vi "App - FileSync Example.vi"() -> ()   [LabVIEW 2020]
uses:
  <userlib>/_NEVSTOP/Communicable State Machine(CSM)/addons/MassData-Parameter/Utility/Def-MassData Status Indicator(Vertical).ctl
  Protocol/Base/Def-FileSyncConfig.ctl
  CSM-FileSync.lvlib
  Protocol/Base/Protocol.lvclass
  Protocol/FTP/FTPProtocol.lvclass
  <userlib>/_NEVSTOP/Communicable State Machine(CSM)/Communicable State Machine.lvlib
  D:/NEVSTOP-LAB-Development/csm-modsets/CSM-ModSets-FileSync/Protocol/Base/Protocol.lvclass
panel:
  in  "MassData Status":T1 {"r" scale=1.0..50000000.0 scale format="%#_6p"; "w" scale=1.0..50000000.0 scale format="%#_6p"}
  in  "stop":bool
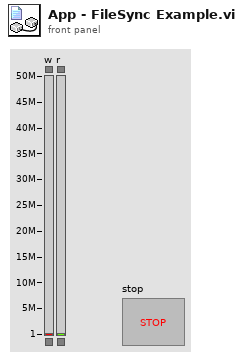
[diagram p1: front panel]
types:
  T1 = typedef "Def-MassData Status Indicator(Vertical).ctl" = cluster{"w":cluster{dbl, dbl}, "r":cluster{dbl, dbl}}
  T2 = typedef "CSM-FileSync.lvlib/Protocol.lvclass/Def-FileSyncConfig.ctl" = cluster{"MonitoringFolder":path, "BackupFolder":path, "autostart":bool, "Backup":bool}
  T3 = cluster{"address":string, "remote port":u16, "userName":string, "passWord":string, "RootDir":string}
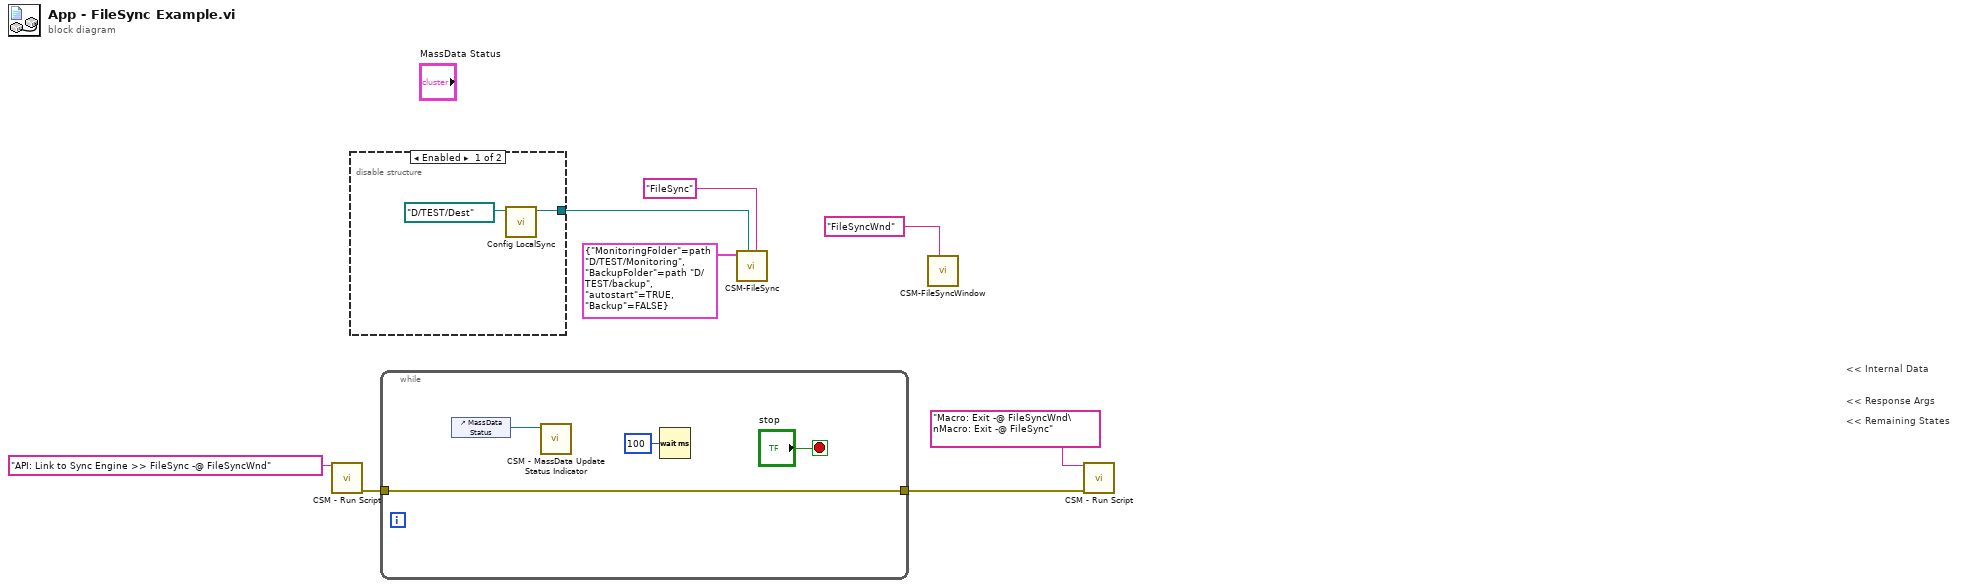
[diagram p0: block diagram]
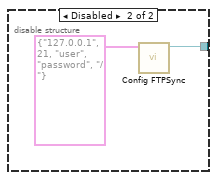
[diagram p2: hidden frame]
diagram:
  # "<< Internal Data"
  # "<< Response Args"
  # "<< Remaining States"
  n1 = call <userlib>:"CSM - Run Script.vi"("CSM Scripts"="API: Link to Sync Engine >> FileSync -@ FileSyncWnd") -> ("error out"=w5:errorcluster)  [unwired: 12 in, 2 out]
  n2 = disable-structure shown="Enabled" {
    disable-tunnel: [w10 w13] -> w7
    frame Enabled {
      n3 = call "Config LocalSync.vi"("Dir"=path "D:/TEST/Dest") -> ("Protocol out"=w10:refnum<class "Protocol.lvclass">)  [unwired: 9 in, 1 out]
    }
    frame Disabled {
      n4 = call "Config FTPSync.vi"("Cluster"=T3 {"address"="127.0.0.1", "remote port"=21, "userName"="user", "passWord"="password", "RootDir"="/"}) -> ("error out"=w11:errorcluster, "FTPProtocol out"=w13:refnum<class "FTPProtocol.lvclass">)  [unwired: 9 in]
    }
  }
  n5 = while {
    tunnel: w5 -> [w14]
    tunnel: [w14] -> w2
    stop <- "stop" stop-if-true
    n6 = control-ref of="MassData Status"() -> (w15:refnum<vi>)
    n7 = call <userlib>:"CSM - MassData Update Status Indicator.vi"("MassData Status Indicator"=w15) -> ()  [unwired: 10 in, 1 out]
    n8 = Wait (ms)(milliseconds to wait=u32 100) -> ()  [unwired: 1 out]
  }
  n9 = call "CSM-FileSync.vi"("Name(FileSync)"="FileSync", "Protocol.lvclass"=w7, "FileSync Configuration"=T2 {"MonitoringFolder"=path "D:/TEST/Monitoring", "BackupFolder"=path "D:/TEST/backup", "autostart"=TRUE, "Backup"=FALSE}) -> ()  [unwired: 8 in, 1 out]
  n10 = call "CSM-FileSyncWindow.vi"("Name(FileSync)"="FileSyncWnd") -> ()  [unwired: 11 in]
  n11 = call <userlib>:"CSM - Run Script.vi"("CSM Scripts"="Macro: Exit -@ FileSyncWnd\nMacro: Exit -@ FileSync", "error in (no error)"=w2) -> ()  [unwired: 11 in, 3 out]
